vi "Test LRS Sums.vi"() -> ()   [LabVIEW 2014]
uses:
  Reusable/General/Math/Fit Exponential Class/Fit Exponential.lvclass
  <vilib>/Analysis/NI_AALPro.lvlib
  <vilib>/Analysis/7linalg.llb/Solve Linear Equations (single right hand).vi
  <vilib>/Analysis/Matrix/NI_Matrix.lvlib
  <vilib>/Analysis/Matrix/Numeric/Conversions/Array To Matrix - RA2.vi
  <vilib>/Analysis/baseanly.llb/Matrix Type of Inverse Matrix.ctl
  <vilib>/Analysis/NI_AALBase.lvlib
  <vilib>/Analysis/7linalg.llb/Real Cholesky Factorization.vi
  <vilib>/Analysis/Matrix/Datatypes/RealMatrix.ctl
panel:
  out "error":i32
  in  "Numeric Indicator":fxp<+,48,48>
  out "output array":fxp<+,64,57>[][](array[numeric]) format="%#.4g"
  out "Cholesky 2":T1
  out "L":fxp<+,64,57>[](array[numeric]) format="%.25g"
  out "Cholesky":T1
  out "Solution Vector 2":dbl[](array[numeric]) format="%.2f"
  out "Solution Vector":dbl[](array[numeric]) format="%.2f"
  out "Waveform Graph":i16[](graph)
  out "x*y 2":dbl format="%#.6f"
  out "Stt":dbl format="%#.6f"
  out "Stt 2":i64 format="%.3e"
  out "St 2":i64
  out "St":dbl
  out "Numeric Control":u32
  out "x-y":u32
  out "Sft 2":i64 format="%.5e"
  out "Sft":i32
  out "StI 2":i64 format="%.5e"
  out "StI":i64
  out "SfI 2":i64 format="%.5e"
  out "SfI":i64
  out "SI 2":i64 format="%.5e"
  out "SI":i64
  out "Sf 2":i32 format="%.5e"
  out "SII 2":i64 format="%.5e"
  out "SII":i64 format="%.6e"
  out "Sf":i64
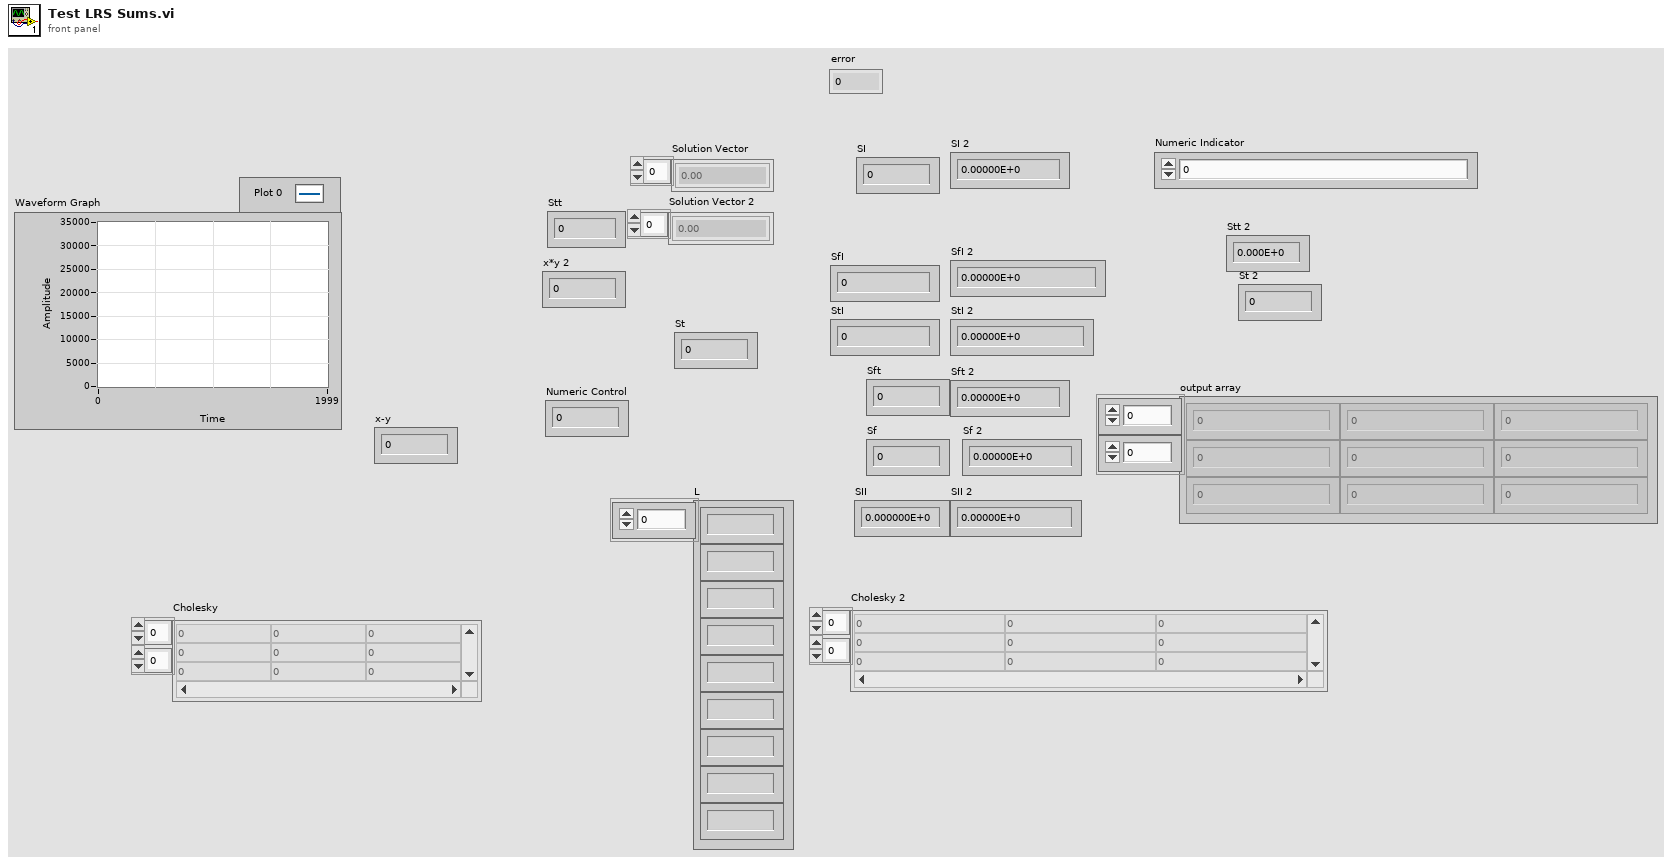
[diagram p1: front panel]
types:
  T1 = typedef "NI_Matrix.lvlib/RealMatrix.ctl" = dbl[][]
  T2 = typedef "NI_AALBase.lvlib/Matrix Type of Inverse Matrix.ctl" = enum32{"General", "Positive Definite", "Lower Triangular", "Upper Triangular"}
  T3 = cluster{"Sf":fxp<+,32,32>, "StI":fxp<+,54,54>, "SI":fxp<+,40,40>, "SfI":fxp<+,54,54>, "SII":fxp<+,64,64>}
  T4 = cluster{"Sf":fxp<+,32,32>, "StI":fxp<+,54,54>, "SI":fxp<+,40,40>, "SfI":fxp<+,54,54>, "SII":fxp<+,64,64>}[]
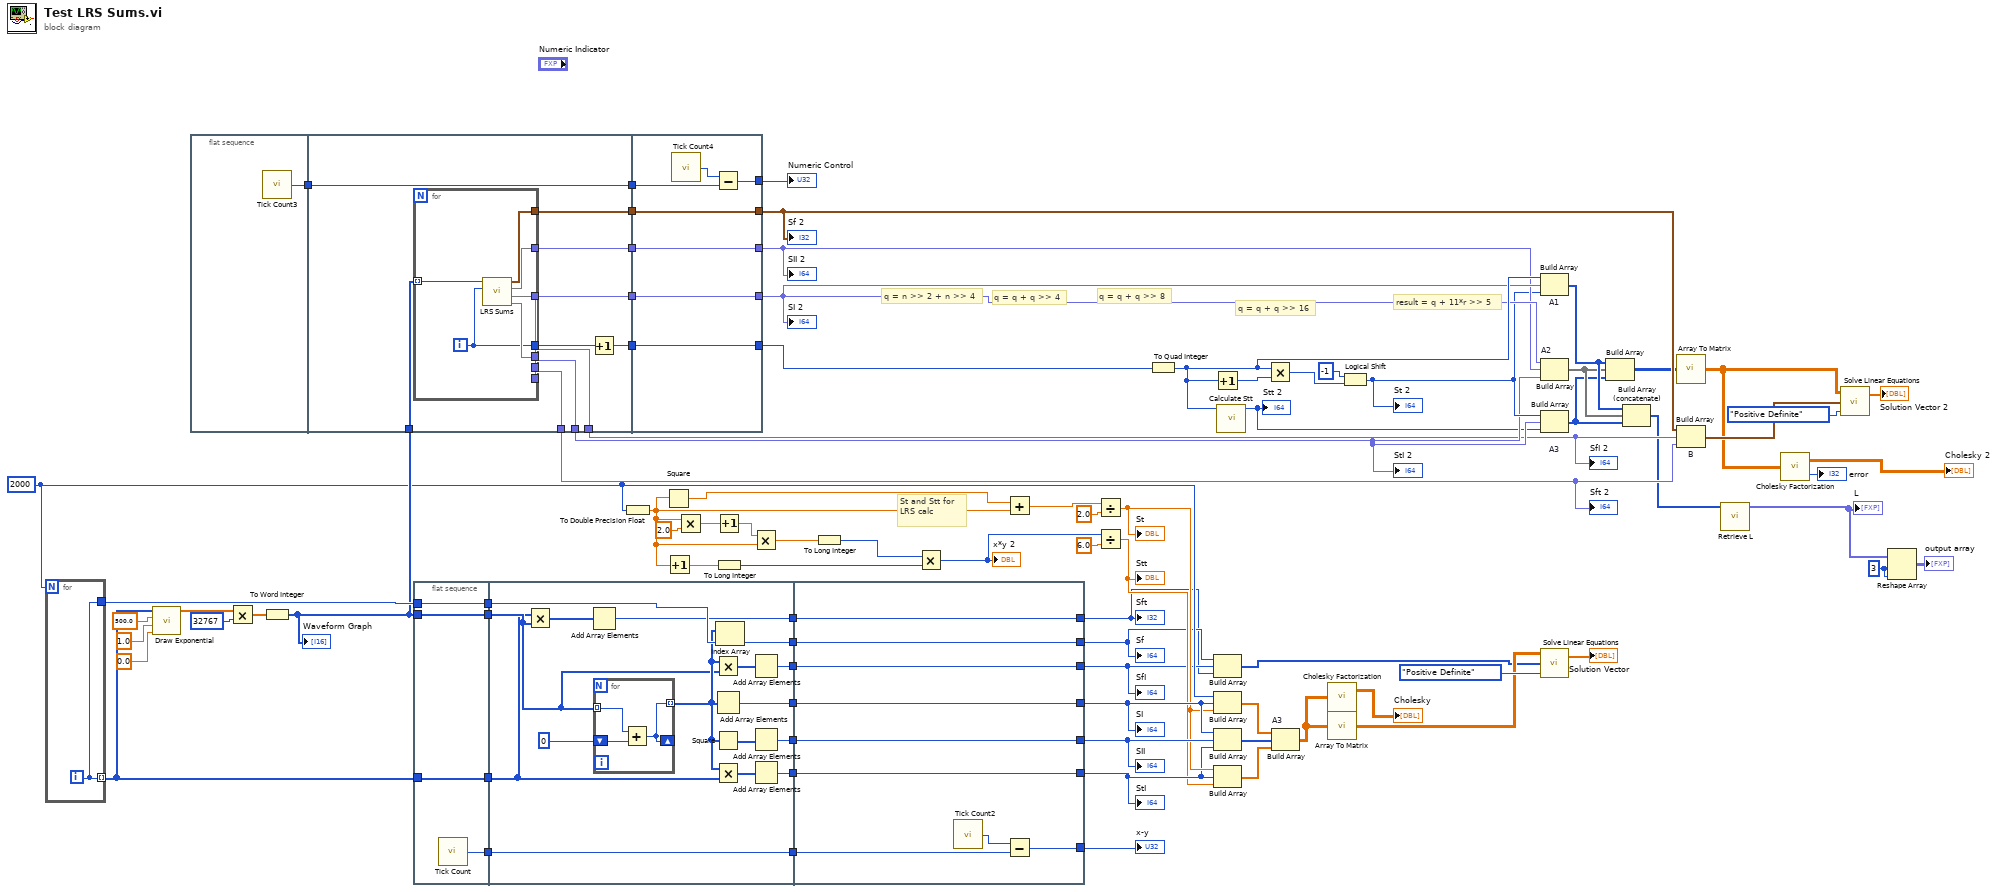
[diagram p0: block diagram]
diagram:
  w3 = 3 ("dimension size")
  w29 = 2000
  # "result = q + 11*r >> 5"
  # "q = q + q >> 16"
  # "q = q + q >> 8"
  # "q = q + q >> 4"
  # "q = n >> 2 + n >> 4"
  # "St and Stt for LRS calc"
  n1 = for {
    N: w29 -> [_]
    tunnel: [w87] -> w86
    tunnel: [w87] -> w55 mode=indexing
    i -> [w87]
  }
  n2 = call "Draw Exponential.vi"("B"=0.0, "A"=1.0, "tau"=500.0, "time"=w55) -> ("ExponentialOut"=w54:dbl[])  [unwired: 7 in]
  n3 = flat-sequence {
    tunnel: [w88] -> w69
    tunnel: [w95] -> w34
    tunnel: [w94] -> w37
    tunnel: w42 -> [w93]
    tunnel: [w92] -> w33
    tunnel: [w98] -> w73
    tunnel: [w97] -> w72
    tunnel: [w96] -> w71
    tunnel: [w91] -> w70
    tunnel: w69 -> [w91]
    tunnel: [w89] -> w67
    tunnel: [w111] -> w40
    tunnel: [w112] -> w39
    tunnel: [w113] -> w35
    tunnel: w73 -> [w113]
    tunnel: w72 -> [w112]
    tunnel: w71 -> [w111]
    tunnel: w70 -> [w109]
    tunnel: [w108] -> w68
    tunnel: [w107] -> w59
    tunnel: w67 -> [w107]
    frame #0 {
      n4 = call "Tick Count3"() -> ("Tick Count(uSec)"=w88:u32)
    }
    frame #1 {
      n5 = for {
        tunnel: w93 -> [w106] mode=indexing
        tunnel: [w104] -> w98
        tunnel: [w105] -> w97
        tunnel: [w103] -> w96
        tunnel: [w102] -> w95
        tunnel: [w101] -> w94
        tunnel: [w100] -> w92
        tunnel: [w99] -> w90
        i -> [w99]
        n6 = call "LRS Sums.vi"("i"=w99, "DataIn"=w106) -> (0:w102, 1:w103, 2:w105, "DataOut"=w104:T3, 4:w101, 6:w100)  [unwired: 4 in]
      }
      n7 = Increment(x=w90) -> (x+1=w89:i32)
    }
    frame #2 {
      n8 = call "Tick Count4"() -> ("Tick Count(uSec)"=w110:u32)
      n9 = Subtract(x=w110, y=w109) -> (x-y=w108:u32)
    }
  }
  n10 = Multiply(x=w54, y=i16 32767) -> (x*y=w52:dbl[])
  n11 = To Word Integer(number=w52) -> (16bit integer=w42:i16[])
  "Waveform Graph" <- w42
  n12 = flat-sequence {
    tunnel: w55 -> [w115]
    tunnel: w42 -> [w116]
    tunnel: w86 -> [w117]
    tunnel: [w117] -> w85
    tunnel: [w116] -> w84
    tunnel: [w115] -> w83
    tunnel: [w114] -> w81
    tunnel: w85 -> [w132]
    tunnel: w84 -> [w128]
    tunnel: w83 -> [w127]
    tunnel: [w124] -> w82
    tunnel: w81 -> [w124]
    tunnel: [w123] -> w80
    tunnel: [w122] -> w79
    tunnel: [w121] -> w78
    tunnel: [w120] -> w77
    tunnel: [w119] -> w76
    tunnel: [w118] -> w75
    tunnel: w82 -> [w144]
    tunnel: w80 -> [w142]
    tunnel: w79 -> [w143]
    tunnel: [w143] -> w27
    tunnel: [w142] -> w18
    tunnel: [w141] -> w28
    tunnel: w78 -> [w141]
    tunnel: [w140] -> w17
    tunnel: w77 -> [w140]
    tunnel: [w139] -> w25
    tunnel: w76 -> [w139]
    tunnel: [w138] -> w16
    tunnel: w75 -> [w138]
    tunnel: [w137] -> w74
    frame #0 {
      n13 = call "Tick Count"() -> ("Tick Count(uSec)"=w114:u32)
    }
    frame #1 {
      n14 = Multiply(x=w127, y=w128) -> (x*y=w126:i32[])
      n15 = Add Array Elements ("SfI")(numeric array=w126) -> (sum=w118:i32)
      n16 = for {
        tunnel: w128 -> [w136] mode=indexing
        tunnel: [w134] -> w130 mode=indexing
        shift-right: [w134] -> _
        shift-left: i64 0 -> [w135]
        n17 = Add(x=w136, y=w135) -> (x+y=w134:i64)
      }
      n18 = Multiply(x=w130, y=w128) -> (x*y=w131:i64[])
      n19 = Add Array Elements ("SII")(numeric array=w130) -> (sum=w121:i64)
      n20 = Square(x=w130) -> (x^2=w125:i64[])
      n21 = Multiply(x=w130, y=w127) -> (x*y=w129:i64[])
      n22 = Index Array(array=w130, index=w132) -> (element=w123:i64)
      n23 = Add Array Elements ("SfI")(numeric array=w131) -> (sum=w120:i64)
      n24 = Add Array Elements ("SII")(numeric array=w125) -> (sum=w122:i64)
      n25 = Add Array Elements ("SfI")(numeric array=w129) -> (sum=w119:i64)
    }
    frame #2 {
      n26 = call "Tick Count2"() -> ("Tick Count(uSec)"=w145:u32)
      n27 = Subtract(x=w145, y=w144) -> (x-y=w137:u32)
    }
  }
  n28 = To Double Precision Float(number=w29) -> (double precision float=w47:dbl)
  n29 = Square(x=w47) -> (x^2=w61:dbl)
  n30 = Increment(x=w47) -> (x+1=w45:dbl)
  n31 = Multiply(x=w47, y=2.0) -> (x*y=w50:dbl)
  n32 = Increment(x=w50) -> (x+1=w49:dbl)
  n33 = To Long Integer(number=w45) -> (32bit integer=w44:i32)
  n34 = Multiply(x=w49, y=w47) -> (x*y=w46:dbl)
  n35 = To Long Integer(number=w46) -> (32bit integer=w43:i32)
  n36 = Multiply(x=w43, y=w44) -> (x*y=w48:i32)
  "x*y 2" <- w48
  n37 = Add(x=w61, y=w47) -> (x+y=w62:dbl)
  n38 = Divide(x=w62, y=2.0) -> (x/y=w26:dbl)
  "St" <- w26
  n39 = Divide(x=w48, y=6.0) -> (x/y=w24:dbl)
  "Stt" <- w24
  n40 = To Quad Integer(1:w59) -> (0:w41:i64)
  n41 = Increment(x=w41) -> (x+1=w60:i64)
  n42 = Build Array(w18, w17, w16) -> (w15:i64[])
  n43 = Build Array(w29, w28, w26) -> (w21:dbl[])
  n44 = Build Array(w28, w27, w25) -> (w20:i64[])
  n45 = Build Array(w26, w25, w24) -> (w19:dbl[])
  n46 = call "Calculate Stt.vi"("N"=w41) -> ("Stt"=w36:i64)  [unwired: 9 in, 1 out]
  "Stt 2" <- w36
  n47 = Multiply(x=w41, y=w60) -> (x*y=w66:i64)
  n48 = Build Array "A3"(w21, w20, w19) -> (w12:dbl[][])
  n49 = call-poly <vilib>:"Cholesky Factorization.vi"("A"=w12) -> ("Cholesky"=→"Cholesky":T1)  [unwired: 1 out]
  n50 = call-poly <vilib>:"Array To Matrix.vi"("Real 2D Array"=w12) -> ("Real Matrix"=w22:T1)
  n51 = Logical Shift(y=i16 -1, x=w66) -> (x << y=w38:i64)
  "St 2" <- w38
  n52 = Build Array "A1"(w41, w40, w38) -> (w10:i64[])
  n53 = Build Array "A2"(w40, w39, w37) -> (w9:void[])
  n54 = Build Array "A3"(w38, w37, w36) -> (w8:i64[])
  n55 = call-poly <vilib>:"Solve Linear Equations.vi"("matrix type"=Matrix_Type_of_Inverse_Matrix."Positive Definite", "Known Vector"=w15, "Input Matrix"=w22) -> ("Solution Vector"=→"Solution Vector":dbl[])  [unwired: 1 out]
  n56 = Build Array(w10, w9, w8) -> (w32:i64[][])
  n57 = Build Array (concatenate)(w10, w9, w8) -> (w7:i64[])
  n58 = call-poly <vilib>:"Array To Matrix.vi"("Real 2D Array"=w32) -> ("Real Matrix"=w6:T1)
  n59 = Build Array "B"(w35, w34, w33) -> (w31:T4)
  n60 = call "Retrieve L.vi"("Matrix In"=w7) -> ("L"=w4:fxp<+,64,57>[])  [unwired: 9 in]
  "L" <- w4
  n61 = call-poly <vilib>:"Cholesky Factorization.vi"("A"=w6) -> ("Cholesky"=→"Cholesky 2":T1, "error"=→"error":i32)
  n62 = call-poly <vilib>:"Solve Linear Equations.vi"("matrix type"=Matrix_Type_of_Inverse_Matrix."Positive Definite", "Known Vector"=w31, "Input Matrix"=w6) -> ("Solution Vector"=→"Solution Vector 2":dbl[])  [unwired: 1 out]
  n63 = Reshape Array(w4, w3, w3) -> (→"output array":fxp<+,64,57>[][])
  "SII 2" <- w39
  "Sf 2" <- w35
  "SI 2" <- w40
  "SfI 2" <- w34
  "StI 2" <- w37
  "Sft 2" <- w33
  "SI" <- w28
  "SII" <- w27
  "Sf" <- w18
  "SfI" <- w17
  "StI" <- w25
  "Sft" <- w16
  "x-y" <- w74
  "Numeric Control" <- w68
